vi "p1230 read bit.vi"(8 "error in (no error)":errorcluster, 9 "pData":u32, 10 "bit":u32, 11 "board_id":u32) -> (0 "error out":errorcluster, 1 "pData out":u32, 3 "function return":u32)   [LabVIEW 2014]
doc: "unsigned int __stdcall p1230_read_bit(unsigned int board_id, unsigned int bit, unsigned int* pData);"
uses:
  PCI1230UTIL.dll
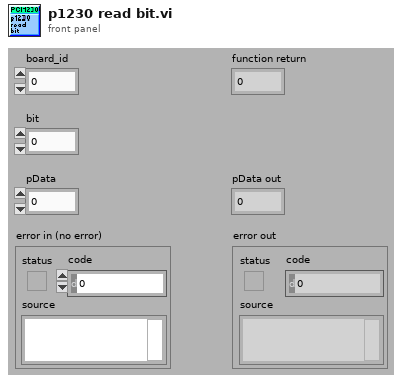
[diagram p1: front panel]
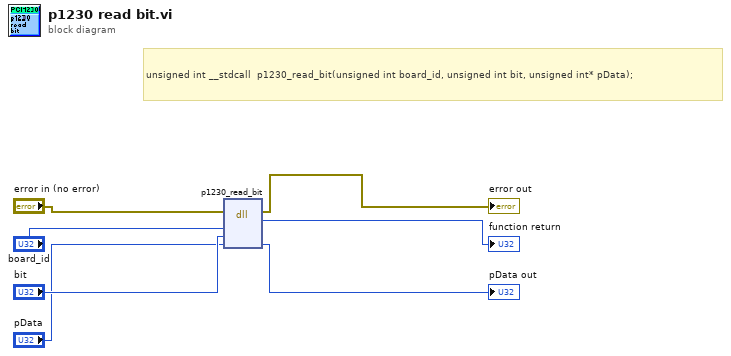
[diagram p0: block diagram]
diagram:
  # "unsigned int __stdcall  p1230_read_bit(unsigned int board_id, unsigned int bit, unsigned int* pData);"
  n1 = dll-call lib="C:/Users/AICTER/Desktop/PCI-1230/PCI1230_VIs/PCI1230UTIL.dll" fn="p1230_read_bit"(error in="error in (no error)", "board_id"="board_id", "bit"="bit", "pData"="pData") -> (error out=→"error out":errorcluster, "return type"=→"function return":u32, "pData"=→"pData out":u32)  [unwired: 4 in, 1 out]
